vi "Close Ref.vi"(8 "error in (no error)":errorcluster, 11 "BK-Precision in":refnum<class "BK-Precision.lvclass">) -> (0 "error out":errorcluster, 3 "BK-Precision out":refnum<class "BK-Precision.lvclass">)   [LabVIEW 2021, in "DC PWS.lvlib" / "BK-Precision.lvclass"]
uses:
  BK-Precision.lvclass
  BK-Precision.lvclass/BK-Precision.ctl
  <instrlib>/BK Precision 911X Series/BK Precision 911X Series.lvlib
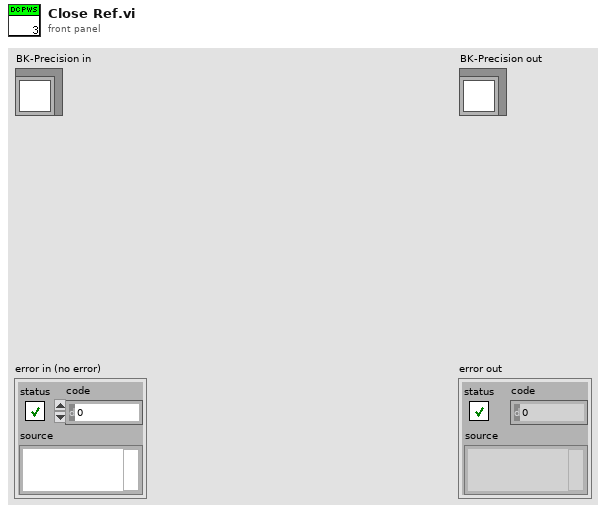
[diagram p1: front panel]
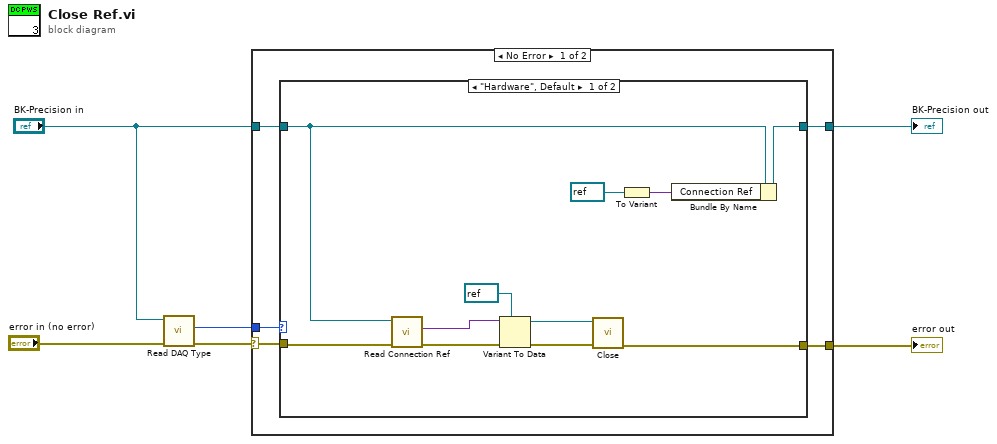
[diagram p0: block diagram]
diagram:
  n1 = call "Read DAQ Type.vi"("error in (no error)"="error in (no error)", "BK-Precision in"="BK-Precision in") -> ("error out"=w5:errorcluster, "Type"=w4:enum16{"Hardware", "Simulation"})  [unwired: 7 in, 1 out]
  n2 = case shown="No Error" w5 {
    selector: w5 -> [w9 w25]
    tunnel: w4 -> [w11 _]
    tunnel: "BK-Precision in" -> [w10 w26]
    tunnel: [w8 w26] -> w2
    tunnel: [w7 w25] -> w1
    frame No Error {
      n3 = case shown="\"Hardware\", Default" w11 {
        tunnel: w10 -> [w16 w24]
        tunnel: w9 -> [w22 w23]
        tunnel: [w14 w24] -> w8
        tunnel: [w15 w23] -> w7
        frame "Hardware", Default {
          n4 = call "Read Connection Ref.vi"("error in (no error)"=w22, "BK-Precision in"=w16) -> ("error out"=w21:errorcluster, "Conn Ref"=w20:variant)  [unwired: 7 in, 1 out]
          n5 = Variant To Data(error in=w21, type=refnum<visa-resource-name> refnum ("VISA resource name"), Variant=w20) -> (data=w18:refnum<visa-resource-name>, error out=w17:errorcluster)
          n6 = call <instrlib>:"Close.vi"("error in (no error)"=w17, "VISA resource name"=w18) -> ("error out"=w15:errorcluster)  [unwired: 9 in]
          n7 = To Variant(anything=refnum<visa-resource-name> refnum ("VISA resource name")) -> (Variant=w12:variant)
          n8 = Bundle By Name(cluster=w16, "Connection Ref"=w12) -> (w14:refnum<class "BK-Precision.lvclass">)
        }
        frame "Simulation" {
        }
      }
    }
    frame Error {
    }
  }
  "error out" <- w1
  "BK-Precision out" <- w2
